vi "Log Error.vi"(8 "error in":errorcluster, 9 "Source":string, 10 "Code":i32, 11 "Error Log Refnum In":refnum<file>) -> (0 "error out":errorcluster, 3 "Error Log Refnum Out":refnum<file>)   [LabVIEW 2017, in "File IO.lvlib"]
uses:
  File IO.lvlib
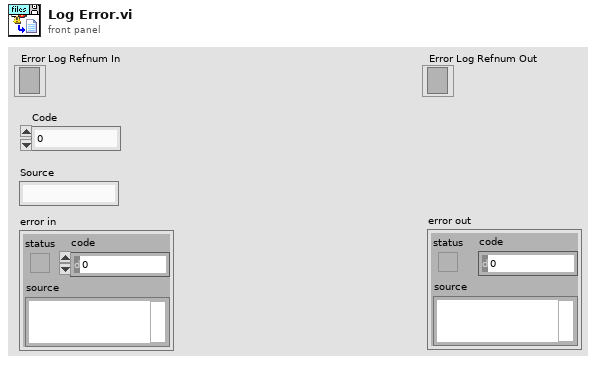
[diagram p1: front panel]
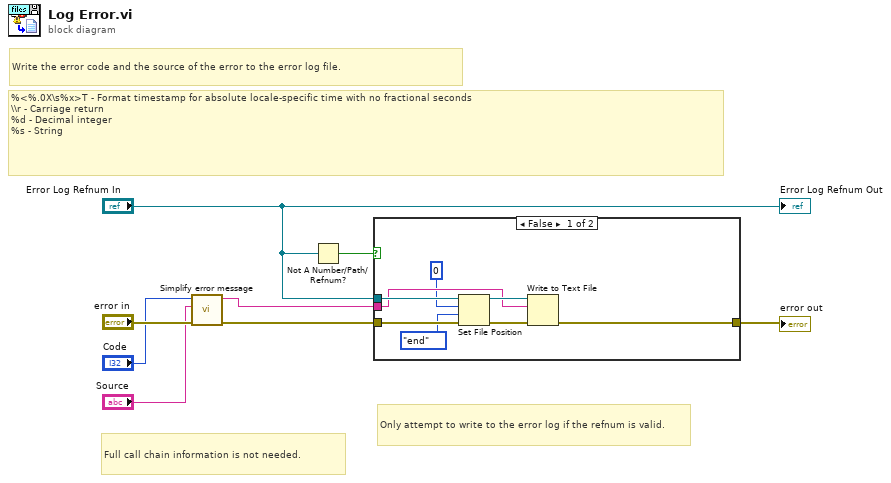
[diagram p0: block diagram]
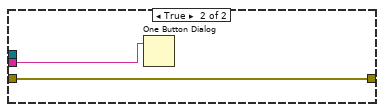
[diagram p2: hidden frame]
diagram:
  # "Full call chain information is not needed."
  # "Only attempt to write to the error log if the refnum is valid."
  # "%<%.0X\\s%x>T - Format timestamp for absolute locale-specific time with no fractional seconds\n\\\\r - Carriage return\n%d - Decimal integer\n%s - String"
  # "Write the error code and the source of the error to the error log file."
  n1 = call "Simplify error message.vi"("error in (no error)"="error in", "Source"="Source", "Code"="Code") -> ("error out"=w8:errorcluster, "String"=w7:string)  [unwired: 7 in]
  n2 = Not A Number/Path/Refnum?(number/path/refnum="Error Log Refnum In") -> (NaN/Path/Refnum?=w4:bool)
  n3 = case shown="False" w4 {
    tunnel: w8 -> [w12 w18]
    tunnel: w7 -> [w11 w17]
    tunnel: [w16 w18] -> w6
    tunnel: "Error Log Refnum In" -> [w14 _]
    frame False {
      n4 = Set File Position(offset (in bytes) (0)=i64 0, refnum=w14, from (0:start)=enum16{"start", "end", "current"}."end", error in=w12) -> (refnum out=w13:refnum<file>, error out=w15:errorcluster)
      n5 = Write to Text File(file (use dialog)=w13, text=w11, error in=w15) -> (error out=w16:errorcluster)  [unwired: 1 in, 2 out]
    }
    frame True {
      n6 = One Button Dialog(message=w17) -> ()  [unwired: 1 in, 1 out]
    }
  }
  "error out" <- w6
  "Error Log Refnum Out" <- "Error Log Refnum In"
